vi "Address Split.vi"(11 "address":u16) -> (0 "wl_addr":u32, 1 "wl_ext_sel":u32, 2 "sl_addr":u32, 3 "sl_ext_sel":u32)   [LabVIEW 2019]
panel:
  out "wl_addr_bool":bool[](array[boolean])
  out "sl_addr_bool":bool[](array[boolean])
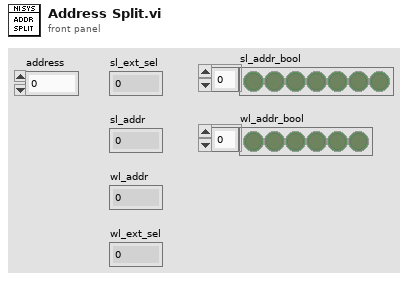
[diagram p1: front panel]
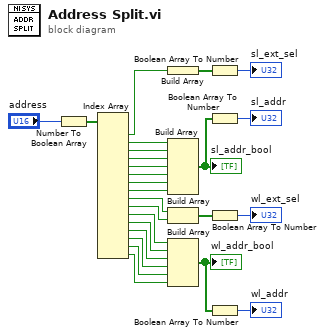
[diagram p0: block diagram]
diagram:
  n1 = Number To Boolean Array(number="address") -> (Boolean array=w7:bool[])
  n2 = Index Array(array=w7) -> (element #1=w5:bool, element #2=w8:bool, element #3=w9:bool, element #4=w10:bool, element #5=w11:bool, element #6=w12:bool, element #7=w13:bool, element #8=w14:bool, element #9=w15:bool, element #10=w16:bool, element #11=w17:bool, element #12=w18:bool, element #13=w19:bool, element #14=w20:bool, element #15=w21:bool, element #16=w22:bool)  [unwired: 16 in]
  n3 = Build Array(w5) -> (w4:bool[])
  n4 = Build Array(w8, w9, w10, w11, w12, w13, w14) -> (w1:bool[])
  "sl_addr_bool" <- w1
  n5 = Build Array(w15, w16) -> (w23:bool[])
  n6 = Build Array(w17, w18, w19, w20, w21, w22) -> (w2:bool[])
  "wl_addr_bool" <- w2
  n7 = Boolean Array To Number(Boolean array=w4) -> (number=→"sl_ext_sel":u32)
  n8 = Boolean Array To Number(Boolean array=w1) -> (number=→"sl_addr":u32)
  n9 = Boolean Array To Number(Boolean array=w23) -> (number=→"wl_ext_sel":u32)
  n10 = Boolean Array To Number(Boolean array=w2) -> (number=→"wl_addr":u32)
